vi "Write parameter.vi"(8 "error in (no error)":errorcluster, 10 "Socket option":T1=enum."ZMQ_SWAP", 11 "Socket2 in":refnum<class "Socket.lvclass">) -> (0 "error out":errorcluster, 3 "Socket2 out":refnum<class "Socket.lvclass">)   [LabVIEW 2018, in "Socket.lvclass"]
uses:
  Socket.lvclass
  <vilib>/addons/zeromq/socket_options.ctl
  Socket.lvclass/Socket.ctl
  <vilib>/addons/zeromq/zeromq.lvlib
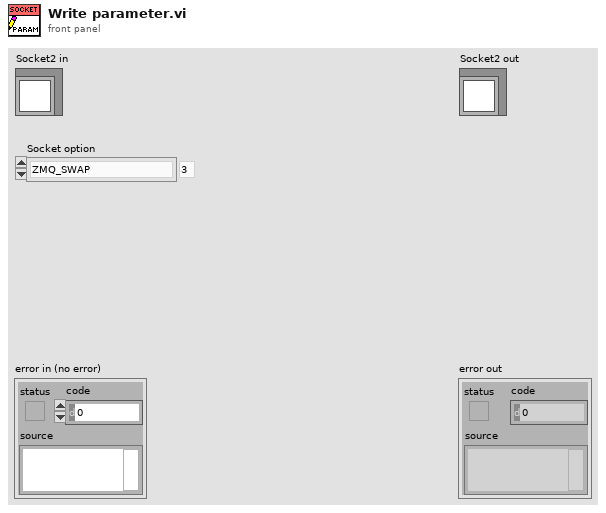
[diagram p1: front panel]
types:
  T1 = typedef "zeromq.lvlib/socket_options.ctl" = enum8{"NONE", "ZMQ_HWM", "<2>", "ZMQ_SWAP", "ZMQ_AFFINITY", "ZMQ_ROUTING_ID", "ZMQ_SUBSCRIBE", "ZMQ_UNSUBSCRIBE", "ZMQ_RATE", "ZMQ_RECOVERY_IVL", "ZMQ_MCAST_LOOP", "ZMQ_SNDBUF", "ZMQ_RCVBUF", "ZMQ_RCVMORE", "ZMQ_FD", "ZMQ_EVENTS", "ZMQ_TYPE", "ZMQ_LINGER", "ZMQ_RECONNECT_IVL", "ZMQ_BACKLOG", "ZMQ_RECOVERY_IVL_MSEC", "ZMQ_RECONNECT_IVL_MAX", "ZMQ_MAXMSGSIZE", "ZMQ_SNDHWM", "ZMQ_RCVHWM", "ZMQ_MULTICAST_HOPS", "<26>", "ZMQ_RCVTIMEO", "ZMQ_SNDTIMEO", "<29>", "<30>", "ZMQ_IPV4ONLY", "ZMQ_LAST_ENDPOINT", "ZMQ_ROUTER_MANDATORY", "ZMQ_TCP_KEEPALIVE", "ZMQ_TCP_KEEPALIVE_CNT", "ZMQ_TCP_KEEPALIVE_IDLE", "ZMQ_TCP_KEEPALIVE_INTVL", "ZMQ_TCP_ACCEPT_FILTER", "ZMQ_IMMEDIATE", "ZMQ_XPUB_VERBOSE", "ZMQ_ROUTER_RAW", "ZMQ_IPV6", "ZMQ_MECHANISM", "ZMQ_PLAIN_SERVER", "ZMQ_PLAIN_USERNAME", "ZMQ_PLAIN_PASSWORD", "ZMQ_CURVE_SERVER", "ZMQ_CURVE_PUBLICKEY", "ZMQ_CURVE_SECRETKEY", "ZMQ_CURVE_SERVERKEY", "ZMQ_PROBE_ROUTER", "ZMQ_REQ_CORRELATE", "ZMQ_REQ_RELAXED", "ZMQ_CONFLATE", "ZMQ_ZAP_DOMAIN", "ZMQ_ROUTER_HANDOVER", "ZMQ_TOS", "ZMQ_IPC_FILTER_PID", "ZMQ_IPC_FILTER_UID", "ZMQ_IPC_FILTER_GID", "ZMQ_CONNECT_ROUTING_ID", "ZMQ_GSSAPI_SERVER", "ZMQ_GSSAPI_PRINCIPAL", "ZMQ_GSSAPI_SERVICE_PRINCIPAL", "ZMQ_GSSAPI_PLAINTEXT", "ZMQ_HANDSHAKE_IVL", "<67>", "ZMQ_SOCKS_PROXY", "ZMQ_XPUB_NODROP", "ZMQ_BLOCKY", "ZMQ_XPUB_MANUAL", "ZMQ_XPUB_WELCOME_MSG", "ZMQ_STREAM_NOTIFY", "ZMQ_INVERT_MATCHING", "ZMQ_HEARTBEAT_IVL", "ZMQ_HEARTBEAT_TTL", "ZMQ_HEARTBEAT_TIMEOUT", "ZMQ_XPUB_VERBOSER", "ZMQ_CONNECT_TIMEOUT", "ZMQ_TCP_MAXRT", "ZMQ_THREAD_SAFE", "<82>", "<83>", "ZMQ_MULTICAST_MAXTPDU", "ZMQ_VMCI_BUFFER_SIZE", "ZMQ_VMCI_BUFFER_MIN_SIZE", "ZMQ_VMCI_BUFFER_MAX_SIZE", "ZMQ_VMCI_CONNECT_TIMEOUT", "ZMQ_USE_FD", "ZMQ_GSSAPI_PRINCIPAL_NAMETYPE", "ZMQ_GSSAPI_SERVICE_PRINCIPAL_NAMETYPE", "ZMQ_BINDTODEVICE", "ZMQ_ZAP_ENFORCE_DOMAIN", "ZMQ_LOOPBACK_FASTPATH", "ZMQ_METADATA", "ZMQ_MULTICAST_LOOP", "ZMQ_ROUTER_NOTIFY"}
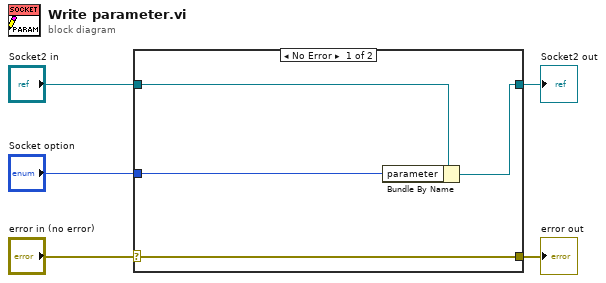
[diagram p0: block diagram]
diagram:
  n1 = case shown="No Error" "error in (no error)" {
    selector: "error in (no error)" -> [w9 w10]
    tunnel: [w9 w10] -> w4
    tunnel: [w7 w11] -> w2
    tunnel: "Socket2 in" -> [w8 w11]
    tunnel: "Socket option" -> [w6 _]
    frame No Error {
      n2 = Bundle By Name(cluster=w8, "parameter"=w6) -> (w7:refnum<class "Socket.lvclass">)
    }
    frame Error {
    }
  }
  "error out" <- w4
  "Socket2 out" <- w2
